vi "weather_parser_nws.vi"() -> ()   [LabVIEW 2011]
uses:
  <vilib>/Utility/miscctls.llb/LVBoundsTypeDef.ctl
  <vilib>/httpClient/LabVIEWHTTPClient.lvlib
panel:
  out "Local IP":string
  out "Warning data":string
  in  "Satellite":bool
  in  "stop 2":bool
  out "Downloaded Picture 2":picture
  out "time string":string
  out "Daylight":picture
  out "Global IP":string
  out "DEFCON":picture
  in  "stop":bool
  out "Downloaded Picture":picture
  out "Alerts":string
  out "Conditions:":string
  out "Wind:":string
  out "Humidity:":string
  out "Temperature:":string
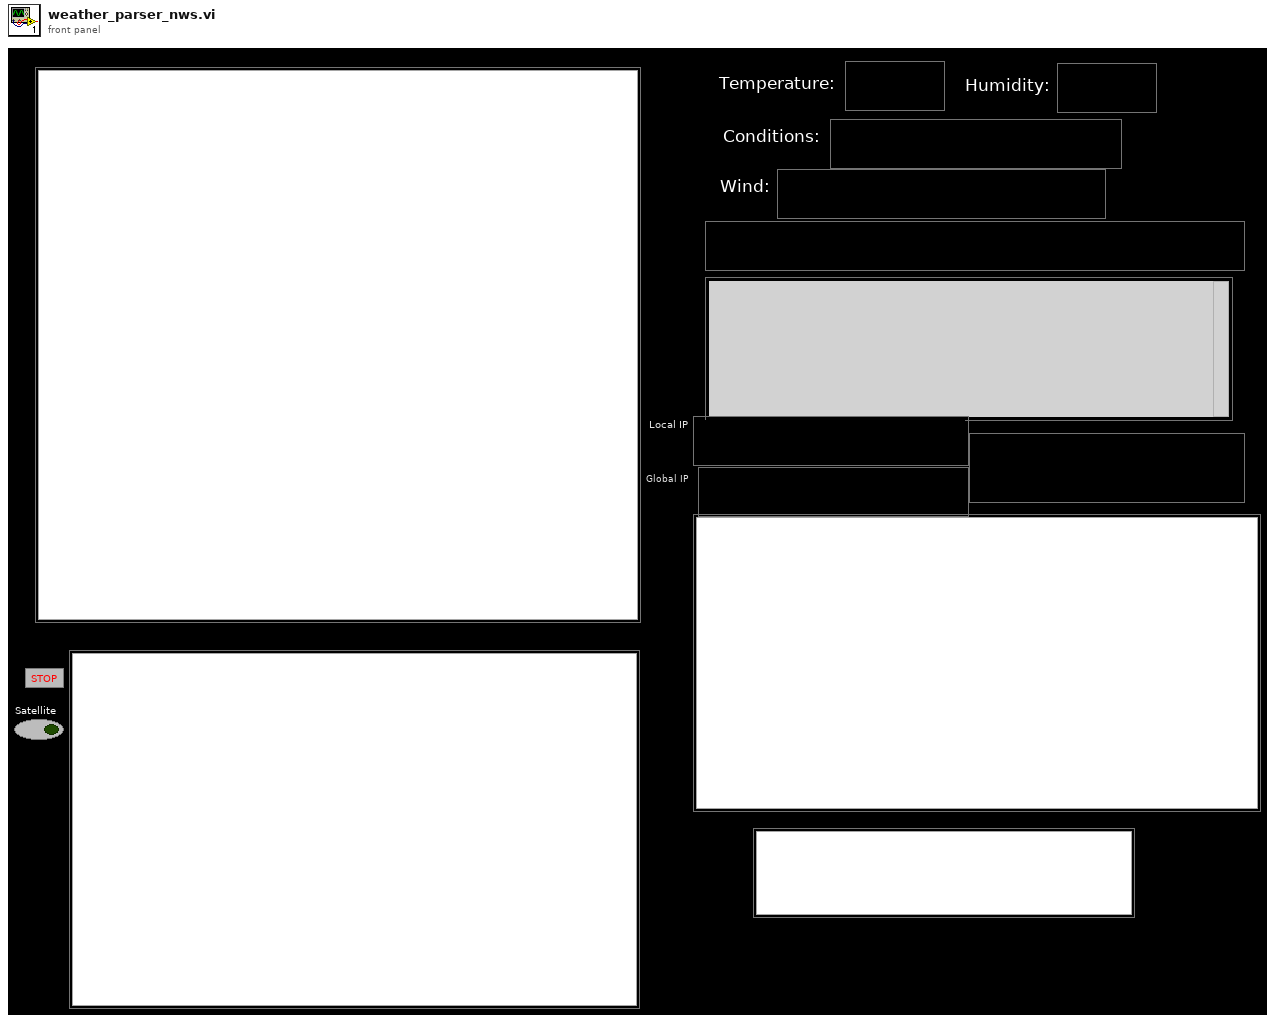
[diagram p1: front panel]
types:
  T1 = typedef "LVBoundsTypeDef.ctl" = cluster{"Width":u32, "Height":u32}
  T2 = typedef "imagedata.ctl" = cluster{"image type":i32, "image depth":i32, "image":u8[], "mask":u8[], "colors":u32[], "Rectangle":cluster{"left":i16, "top":i16, "right":i16, "bottom":i16}}
  T3 = cluster{"left":i16, "top":i16, "right":i16, "bottom":i16}
  T4 = enum16{"open", "replace", "create", "open or create", "replace or create", "replace or create with confirmation"}
  T5 = typedef "LVAllMonitorsDisplayTypeDef.ctl" = cluster{"Bounds":cluster{"Left":i16, "Top":i16, "Right":i16, "Bottom":i16}, "Depth":i16}[]
  T6 = cluster{"Bounds":cluster{"Left":i16, "Top":i16, "Right":i16, "Bottom":i16}, "Depth":i16}
  T7 = cluster{"Left":i16, "Top":i16, "Right":i16, "Bottom":i16}
  T8 = cluster{"Width":u16, "Style":enum32{"Solid", "Dash", "Dot", "DashDot", "DashDotDot"}}
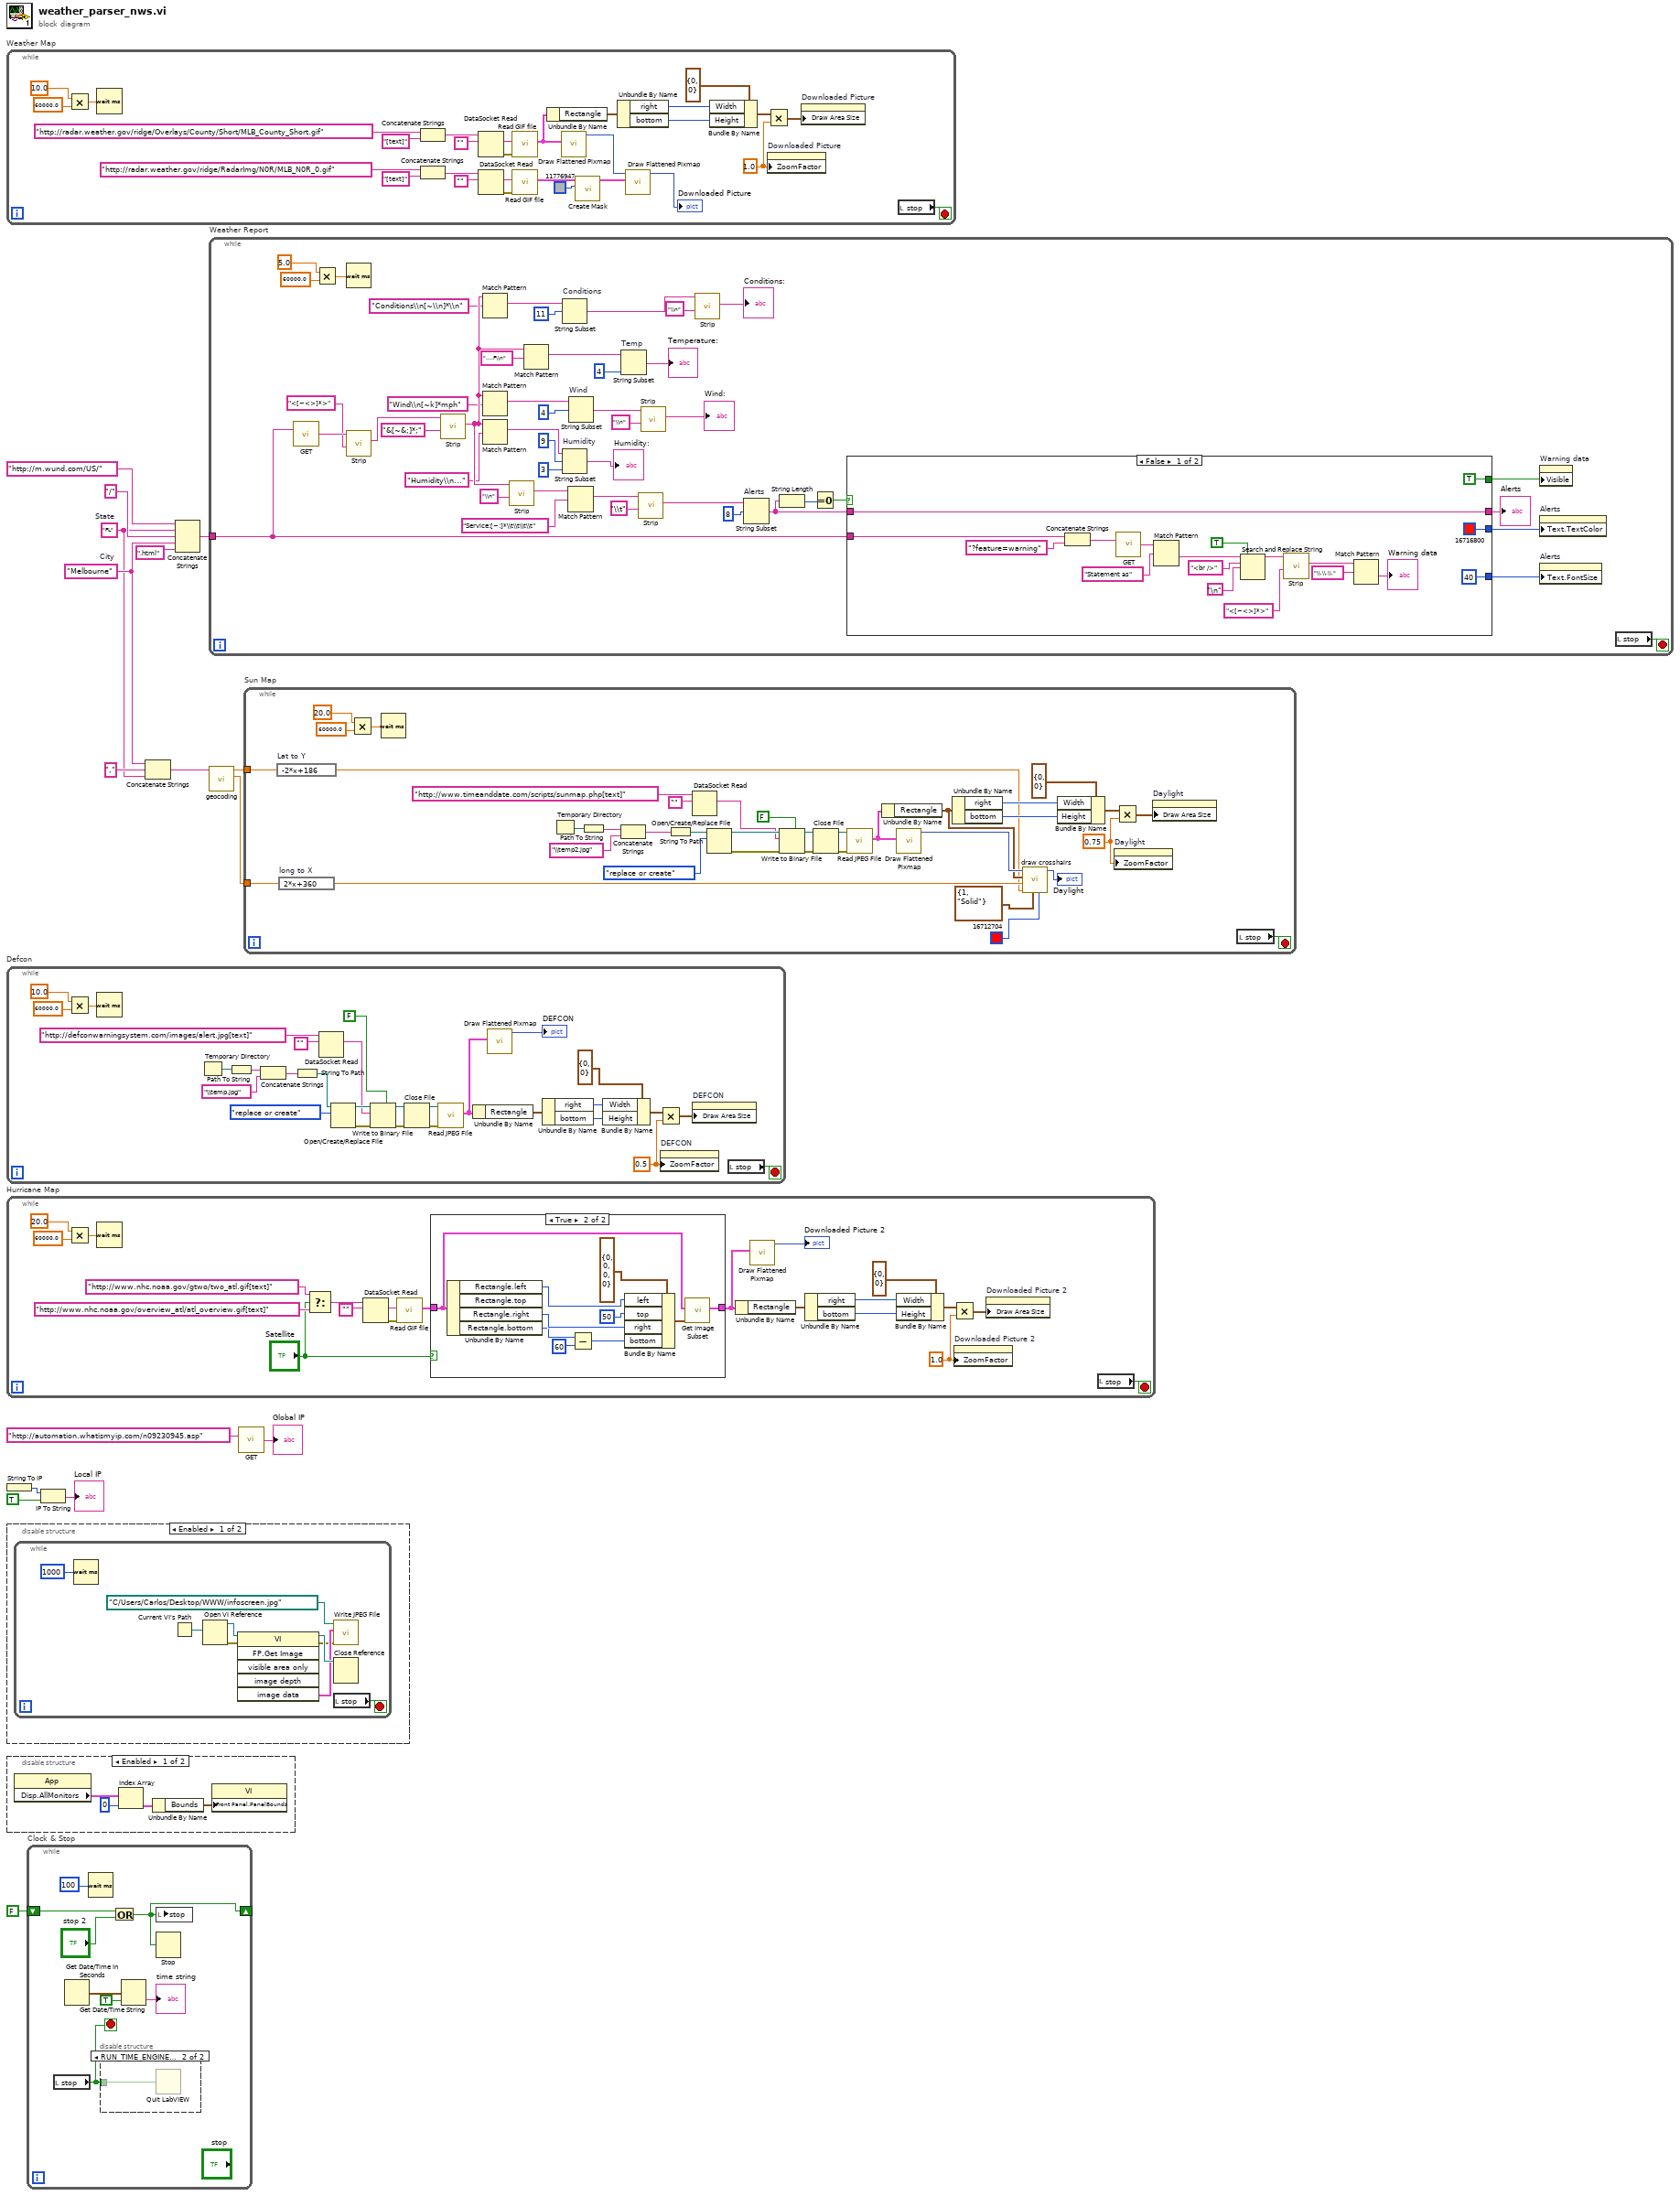
[diagram p0: block diagram]
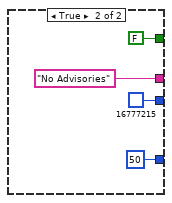
[diagram p3: hidden frame]
diagram:
  w10 = "FL"  # State
  w12 = "Melbourne"  # City
  n1 = while "Weather Map" {
    stop <- w17 stop-if-true
    w27 = sgl 1.0 ("Zoom Factor")
    n2 = Multiply(x=10.0, y=60000.0) -> (x*y=w20:dbl)
    n3 = Wait (ms)(milliseconds to wait=w20) -> ()  [unwired: 1 out]
    n4 = Concatenate Strings("http://radar.weather.gov/ridge/Overlays/County/Short/MLB_County_Short.gif" ("string"), "[text]" ("string")) -> (w24:string)
    n5 = Concatenate Strings("http://radar.weather.gov/ridge/RadarImg/N0R/MLB_N0R_0.gif" ("string"), "[text]" ("string")) -> (w38:string)
    n6 = DataSocket Read(10:"", 11:w24) -> (0:w22:errorcluster, 2:w23:string)  [unwired: 3 in, 5 out]
    n7 = DataSocket Read(10:"", 11:w38) -> (0:w21:errorcluster, 2:w37:string)  [unwired: 3 in, 5 out]
    n8 = call "Read GIF file.vi"("error in (no error)"=w22, "String"=w23) -> ("image data"=w42:T2)  [unwired: 8 in, 1 out]
    n9 = call "Read GIF file.vi"("error in (no error)"=w21, "String"=w37) -> ("image data"=w41:T2)  [unwired: 8 in, 1 out]
    n10 = Unbundle By Name(w42) -> ("Rectangle"=w32:T3)
    n11 = call <vilib>:"Draw Flattened Pixmap.vi"("image data"=w42) -> ("new picture"=w43:picture)  [unwired: 3 in, 5 out]
    n12 = call <vilib>:"Create Mask.vi"("Mask Color (Black)"=u32 11776947, "image data"=w41) -> ("image data"=w45:T2)  [unwired: 9 in]
    n13 = Unbundle By Name(w32) -> ("right"=w30:i16, "bottom"=w29:i16)
    n14 = call <vilib>:"Draw Flattened Pixmap.vi"("image data"=w45, "picture"=w43) -> ("new picture"=→"Downloaded Picture":picture)  [unwired: 2 in, 5 out]
    n15 = Bundle By Name(cluster=T1 {"Width"=0, "Height"=0} ("Draw Area Size"), "Width"=w30, "Height"=w29) -> (w28:T1)
    n16 = Multiply(x=w28, y=w27) -> (x*y=w26:cluster{"Width":sgl, "Height":sgl})
    n17 = property on="Downloaded Picture" class="Pict"("ZoomFactor"=w27) -> ()  [unwired: 2 in, 2 out]
    n18 = property on="Downloaded Picture" class="Pict"("Draw Area Size"=w26) -> ()  [unwired: 2 in, 2 out]
    n19 = local read "stop"() -> (w17:bool)
  }
  n20 = while "Defcon" {
    stop <- w49 stop-if-true
    w50 = sgl 0.5 ("Zoom Factor")
    n21 = Multiply(x=10.0, y=60000.0) -> (x*y=w48:dbl)
    n22 = Wait (ms)(milliseconds to wait=w48) -> ()  [unwired: 1 out]
    n23 = Temporary Directory() -> (w71:path)
    n24 = Path To String(path=w71) -> (string=w72:string)
    n25 = Concatenate Strings(w72, "\\temp.jpg" ("string")) -> (w74:string)
    n26 = String To Path(string=w74) -> (path=w65:path)
    n27 = DataSocket Read(10:"", 11:"http://defconwarningsystem.com/images/alert.jpg[text]" ("connection in")) -> (2:w66:string)  [unwired: 3 in, 6 out]
    n28 = Open/Create/Replace File(file path (use dialog)=w65, operation (0:open)=T4."replace or create") -> (refnum out=w67:refnum<file>, error out=w62:errorcluster)  [unwired: 4 in, 1 out]
    n29 = Write to Binary File(file (use dialog)=w67, data=w66, error in=w62, 5:FALSE ("prepend array or string size? (T)")) -> (refnum out=w64:refnum<file>, error out=w63:errorcluster)  [unwired: 2 in, 1 out]
    n30 = Close File(refnum=w64, error in=w63) -> (path=w60:path, error out=w59:errorcluster)
    n31 = call <vilib>:"Read JPEG File.vi"("error in (no error)"=w59, "path to JPEG file"=w60) -> ("image data"=w52:T2)  [unwired: 7 in, 2 out]
    n32 = Unbundle By Name(w52) -> ("Rectangle"=w57:T3)
    n33 = call <vilib>:"Draw Flattened Pixmap.vi"("image data"=w52) -> ("new picture"=→"DEFCON":picture)  [unwired: 3 in, 5 out]
    n34 = Unbundle By Name(w57) -> ("right"=w55:i16, "bottom"=w54:i16)
    n35 = Bundle By Name(cluster=T1 {"Width"=0, "Height"=0} ("Draw Area Size"), "Width"=w55, "Height"=w54) -> (w53:T1)
    n36 = Multiply(x=w53, y=w50) -> (x*y=w51:cluster{"Width":sgl, "Height":sgl})
    n37 = property on="DEFCON" class="Pict"("ZoomFactor"=w50) -> ()  [unwired: 2 in, 2 out]
    n38 = property on="DEFCON" class="Pict"("Draw Area Size"=w51) -> ()  [unwired: 2 in, 2 out]
    n39 = local read "stop"() -> (w49:bool)
  }
  n40 = while "Hurricane Map" {
    stop <- w78 stop-if-true
    w92 = sgl 1.0 ("Zoom Factor")
    n41 = Multiply(x=20.0, y=60000.0) -> (x*y=w77:dbl)
    n42 = Wait (ms)(milliseconds to wait=w77) -> ()  [unwired: 1 out]
    n43 = Select(t="http://www.nhc.noaa.gov/gtwo/two_atl.gif[text]", s="Satellite", f="http://www.nhc.noaa.gov/overview_atl/atl_overview.gif[text]") -> (s? t:f=w85:string)
    n44 = DataSocket Read(10:"", 11:w85) -> (0:w95:errorcluster, 2:w94:string)  [unwired: 3 in, 5 out]
    n45 = call "Read GIF file.vi"("error in (no error)"=w95, "String"=w94) -> ("image data"=w81:T2)  [unwired: 8 in, 1 out]
    n46 = case shown="True" "Satellite" {
      tunnel: w81 -> [w96 w105]
      tunnel: [w96 w106] -> w80
      frame False {
      }
      frame True {
        n47 = Unbundle By Name(w105) -> ("Rectangle.left"=w102:i16, "Rectangle.right"=w101:i16, "Rectangle.bottom"=w99:i16)  [unwired: 1 out]
        n48 = Subtract(x=w99, y=i16 60 ("bottom")) -> (x-y=w97:i16)
        n49 = Bundle By Name(cluster=T3 {"left"=0, "top"=0, "right"=0, "bottom"=0} ("subset rect"), "left"=w102, "top"=i16 50, "right"=w101, "bottom"=w97) -> (w104:T3)
        n50 = call <vilib>:"Get Image Subset.vi"("subset rect"=w104, "image data"=w105) -> ("image subset"=w106:T2)  [unwired: 4 in, 1 out]
      }
    }
    n51 = Unbundle By Name(w80) -> ("Rectangle"=w88:T3)
    n52 = call <vilib>:"Draw Flattened Pixmap.vi"("image data"=w80) -> ("new picture"=→"Downloaded Picture 2":picture)  [unwired: 3 in, 5 out]
    n53 = Unbundle By Name(w88) -> ("right"=w89:i16, "bottom"=w90:i16)
    n54 = Bundle By Name(cluster=T1 {"Width"=0, "Height"=0} ("Draw Area Size"), "Width"=w89, "Height"=w90) -> (w91:T1)
    n55 = Multiply(x=w91, y=w92) -> (x*y=w93:cluster{"Width":sgl, "Height":sgl})
    n56 = property on="Downloaded Picture 2" class="Pict"("ZoomFactor"=w92) -> ()  [unwired: 2 in, 2 out]
    n57 = property on="Downloaded Picture 2" class="Pict"("Draw Area Size"=w93) -> ()  [unwired: 2 in, 2 out]
    n58 = local read "stop"() -> (w78:bool)
  }
  n59 = String To IP() -> (0:w3:u32)  [unwired: 1 in]
  n60 = disable-structure shown="Enabled" {
    frame Enabled {
      n61 = while {
        stop <- w108 stop-if-true
        n62 = Wait (ms)(milliseconds to wait=u32 1000) -> ()  [unwired: 1 out]
        n63 = Current VI's Path() -> (path=w115:path)
        n64 = Open VI Reference(vi path=w115) -> (vi reference=w114:refnum<vi>, error out=w113:errorcluster)  [unwired: 5 in]
        n65 = invoke class="VI" method="FP.Get Image"(reference=w114, error in=w113) -> (reference out=w112:refnum<vi>, error out=w109:errorcluster, "image data"=w111:T2)  [unwired: 4 in, 3 out]
        n66 = call <vilib>:"Write JPEG File.vi"("error in (no error)"=w109, "image data"=w111, "path to JPEG file"=path "C:/Users/Carlos/Desktop/WWW/infoscreen.jpg") -> ()  [unwired: 7 in, 2 out]
        n67 = Close Reference(reference=w112) -> ()  [unwired: 1 in, 1 out]
        n68 = local read "stop"() -> (w108:bool)
      }
    }
    frame Disabled {
    }
  }
  n69 = disable-structure shown="Enabled" {
    frame Enabled {
      n70 = property class="App"() -> ("Disp.AllMonitors"=w118:T5)  [unwired: 2 in, 2 out]
      n71 = Index Array(array=w118, index=0) -> (element=w117:T6)
      n72 = Unbundle By Name(w117) -> ("Bounds"=w119:T7)
      n73 = property class="VI"("Front Panel.PanelBounds"=w119) -> ()  [unwired: 2 in, 2 out]
    }
    frame Disabled {
    }
  }
  n74 = while "Clock & Stop" {
    shift-right: [w121] -> _
    shift-left: FALSE -> [w122]
    stop <- w120 stop-if-true
    n75 = local read "stop"() -> (w120:bool)
    n76 = Get Date/Time In Seconds() -> (seconds since 1Jan1904=w125:timestamp)
    n77 = Wait (ms)(milliseconds to wait=u32 100) -> ()  [unwired: 1 out]
    n78 = disable-structure shown="RUN_TIME_ENGINE==True" {
      disable-tunnel: w120 -> [_ w128]
      frame condition #0 (active) {
      }
      frame condition #1 {
        n79 = Quit LabVIEW(quit? (T)=w128) -> ()
      }
    }
    n80 = Or(x=w122, y="stop 2") -> (x .or. y?=w121:bool)
    n81 = Get Date/Time String(seconds (now)=w125, want seconds? (F)=TRUE) -> (time string=→"time string":string)  [unwired: 1 in, 1 out]
    n82 = local write "stop"(w121) -> ()
    n83 = Stop(stop? (T)=w121) -> ()
  }
  n84 = IP To String(1:TRUE ("dot notation? (F)"), 2:w3) -> (0:→"Local IP":string)
  n85 = Concatenate Strings(w12, "," ("string"), w10) -> (w9:string)
  n86 = Concatenate Strings("http://m.wund.com/US/" ("url"), w10, "/" ("string"), w12, ".html" ("string")) -> (w13:string)
  n87 = while "Weather Report" {
    tunnel: w13 -> [w173]
    stop <- w132 stop-if-true
    n88 = call <vilib>:"GET.vi"("url"=w173) -> ("body"=w172:string)  [unwired: 11 in, 3 out]
    n89 = Multiply(x=5.0, y=60000.0) -> (x*y=w131:dbl)
    n90 = Wait (ms)(milliseconds to wait=w131) -> ()  [unwired: 1 out]
    n91 = call "Strip.vi"("Regex"="<[~<>]*>", "Input String"=w172) -> ("Result String"=w150:string)  [unwired: 9 in]
    n92 = call "Strip.vi"("Regex"="&[~&;]*;", "Input String"=w150) -> ("Result String"=w156:string)  [unwired: 9 in]
    n93 = Match Pattern(string=w156, regular expression="Conditions\\n[~\\n]*\\n") -> (match substring=w146:string)  [unwired: 1 in, 3 out]
    n94 = Match Pattern(string=w156, regular expression="Wind\\n[~k]*mph") -> (match substring=w143:string)  [unwired: 1 in, 3 out]
    n95 = Match Pattern(string=w156, regular expression="Humidity\\n...") -> (match substring=w139:string)  [unwired: 1 in, 3 out]
    n96 = call "Strip.vi"("Regex"="\\n", "Input String"=w156) -> ("Result String"=w158:string)  [unwired: 9 in]
    n97 = Match Pattern(string=w156, regular expression="....F\\n") -> (match substring=w136:string)  [unwired: 1 in, 3 out]
    n98 = String Subset "Conditions"(string=w146, offset (0)=11) -> (substring=w153:string)  [unwired: 1 in]
    n99 = String Subset "Humidity"(string=w139, offset (0)=9, length (rest)=3 ("length (rest)")) -> (substring=→"Humidity:":string)
    n100 = Match Pattern(string=w158, regular expression="Service:[~:]*\\t\\t\\t\\t") -> (match substring=w159:string)  [unwired: 1 in, 3 out]
    n101 = String Subset "Wind"(string=w143, offset (0)=4) -> (substring=w151:string)  [unwired: 1 in]
    n102 = String Subset "Temp"(string=w136, length (rest)=4 ("length (rest)")) -> (substring=→"Temperature:":string)  [unwired: 1 in]
    n103 = call "Strip.vi"("Regex"="\\t", "Input String"=w159) -> ("Result String"=w161:string)  [unwired: 9 in]
    n104 = call "Strip.vi"("Regex"="\\n", "Input String"=w151) -> ("Result String"=→"Wind:":string)  [unwired: 9 in]
    n105 = call "Strip.vi"("Regex"="\\n", "Input String"=w153) -> ("Result String"=→"Conditions:":string)  [unwired: 9 in]
    n106 = String Subset "Alerts"(string=w161, offset (0)=8) -> (substring=w169:string)  [unwired: 1 in]
    n107 = String Length(string=w169) -> (length=w167:i32)
    n108 = Equal To 0?(x=w167) -> (x = 0?=w168:bool)
    n109 = case shown="False" w168 {
      tunnel: w169 -> [w191 _]
      tunnel: [w191 "No Advisories" ("Result String")] -> w170
      tunnel: [u32 16716800 u32 16777215] -> w171
      tunnel: w173 -> [w189 _]
      tunnel: [TRUE FALSE] -> w134
      tunnel: [u32 40 u32 50] -> w133
      frame False {
        n110 = Concatenate Strings(w189, "?feature=warning" ("string")) -> (w187:string)
        n111 = call <vilib>:"GET.vi"("url"=w187) -> ("body"=w186:string)  [unwired: 11 in, 3 out]
        n112 = Match Pattern(string=w186, regular expression="Statement as") -> (after substring=w174:string)  [unwired: 1 in, 3 out]
        n113 = Search and Replace String(replace all?=TRUE ("replace all? (F)"), input string=w174, search string="<br />", replace string="\n") -> (result string=w181:string)  [unwired: 4 in, 3 out]
        n114 = call "Strip.vi"("Regex"="<[~<>]*>", "Input String"=w181) -> ("Result String"=w179:string)  [unwired: 9 in]
        n115 = Match Pattern(string=w179, regular expression="\\.\\.\\.") -> (after substring=→"Warning data":string)  [unwired: 1 in, 3 out]
      }
      frame True {
      }
    }
    "Alerts" <- w170
    n116 = property on="Warning data" class="Str"("Visible"=w134) -> ()  [unwired: 2 in, 2 out]
    n117 = property on="Alerts" class="Str"("Text.TextColor"=w171) -> ()  [unwired: 2 in, 2 out]
    n118 = property on="Alerts" class="Str"("Text.FontSize"=w133) -> ()  [unwired: 2 in, 2 out]
    n119 = local read "stop"() -> (w132:bool)
  }
  n120 = call "geocoding.vi"("Location"=w9) -> ("Longitude"=w8:dbl, "Latitude"=w7:dbl)  [unwired: 9 in]
  n121 = call <vilib>:"GET.vi"("url"="http://automation.whatismyip.com/n09230945.asp") -> ("body"=→"Global IP":string)  [unwired: 11 in, 3 out]
  n122 = while "Sun Map" {
    tunnel: w8 -> [w231]
    tunnel: w7 -> [w230]
    stop <- w199 stop-if-true
    w207 = sgl 0.75 ("Zoom Factor")
    n123 = expression code="-2*x+186" "Lat to Y"(w230) -> (w200:dbl)
    n124 = expression code="2*x+360" "long to X"(w231) -> (w201:dbl)
    n125 = Multiply(x=20.0, y=60000.0) -> (x*y=w198:dbl)
    n126 = Wait (ms)(milliseconds to wait=w198) -> ()  [unwired: 1 out]
    n127 = Temporary Directory() -> (w226:path)
    n128 = Path To String(path=w226) -> (string=w227:string)
    n129 = Concatenate Strings(w227, "\\temp2.jpg" ("string")) -> (w229:string)
    n130 = String To Path(string=w229) -> (path=w220:path)
    n131 = DataSocket Read(10:"", 11:"http://www.timeanddate.com/scripts/sunmap.php[text]" ("connection in")) -> (2:w221:string)  [unwired: 3 in, 6 out]
    n132 = Open/Create/Replace File(file path (use dialog)=w220, operation (0:open)=T4."replace or create") -> (refnum out=w222:refnum<file>, error out=w217:errorcluster)  [unwired: 4 in, 1 out]
    n133 = Write to Binary File(file (use dialog)=w222, data=w221, error in=w217, 5:FALSE ("prepend array or string size? (T)")) -> (refnum out=w219:refnum<file>, error out=w218:errorcluster)  [unwired: 2 in, 1 out]
    n134 = Close File(refnum=w219, error in=w218) -> (path=w216:path, error out=w215:errorcluster)
    n135 = call <vilib>:"Read JPEG File.vi"("error in (no error)"=w215, "path to JPEG file"=w216) -> ("image data"=w209:T2)  [unwired: 7 in, 2 out]
    n136 = Unbundle By Name(w209) -> ("Rectangle"=w202:T3)
    n137 = call <vilib>:"Draw Flattened Pixmap.vi"("image data"=w209) -> ("new picture"=w206:picture)  [unwired: 3 in, 5 out]
    n138 = Unbundle By Name(w202) -> ("right"=w212:i16, "bottom"=w211:i16)
    n139 = call "draw crosshairs.vi"("color(black)"=u32 16712704, "pen"=T8 {"Width"=1, "Style"=enum."Solid"}, "Y"=w200, "X"=w201, "Rectangle"=w202, "picture"=w206) -> ("new picture"=→"Daylight":picture)  [unwired: 5 in]
    n140 = Bundle By Name(cluster=T1 {"Width"=0, "Height"=0} ("Draw Area Size"), "Width"=w212, "Height"=w211) -> (w210:T1)
    n141 = property on="Daylight" class="Pict"("ZoomFactor"=w207) -> ()  [unwired: 2 in, 2 out]
    n142 = Multiply(x=w210, y=w207) -> (x*y=w208:cluster{"Width":sgl, "Height":sgl})
    n143 = property on="Daylight" class="Pict"("Draw Area Size"=w208) -> ()  [unwired: 2 in, 2 out]
    n144 = local read "stop"() -> (w199:bool)
  }
